vi "InitializeExpDepsFilesWithActualDeps.vi"() -> ()   [LabVIEW 2023, in "Reusables.lvlib"]
uses:
  Reusables/Reusables.lvlib
  <userlib>/_OpenG.lib/file/file.llb/File Exists - Scalar__ogtk.vi
  <userlib>/_OpenG.lib/file/file.llb/openg_file.lvlib
  <vilib>/Utility/config.llb/NI_LVConfig.lvlib
panel:
  out "error out":errorcluster
  in  "Build Specs Folder Path":path=path "E:/sw-deps-monitor/Source/BuildSpecs"
  in  "error in (no error)":errorcluster
  in  "Source Folder Path":path=path "E:/sw-deps-monitor/Source"
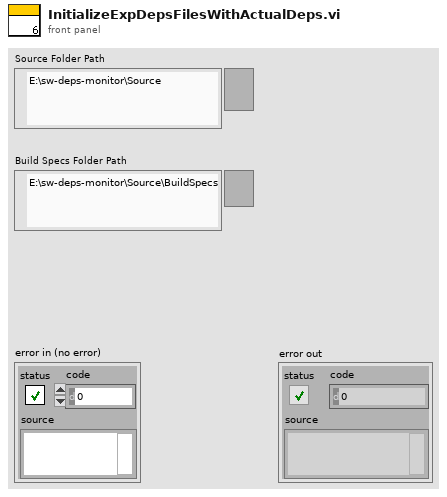
[diagram p1: front panel]
types:
  T1 = typedef "NI_LVConfig.lvlib/Config Data RefNum.ctl" = refnum<k1>
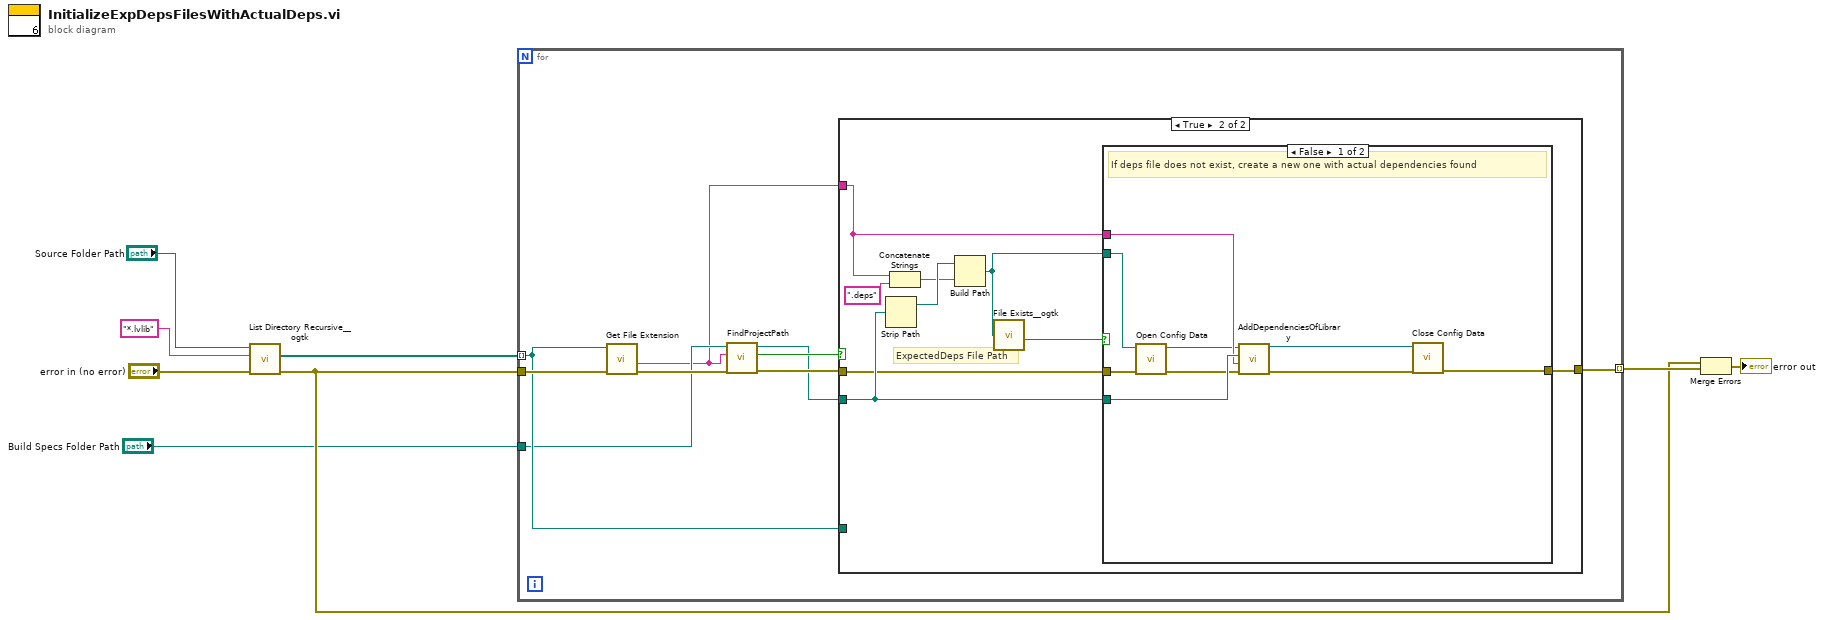
[diagram p0: block diagram]
diagram:
  n1 = call <userlib>:"List Directory Recursive__ogtk.vi"("error in (no error)"="error in (no error)", "pattern"="*.lvlib", "Path"="Source Folder Path") -> ("error out"=w3:errorcluster, "file paths"=w5:path[])  [unwired: 5 in, 2 out]
  n2 = for {
    tunnel: w3 -> [w17]
    tunnel: w5 -> [w15] mode=indexing
    tunnel: "Build Specs Folder Path" -> [w13]
    tunnel: [w16] -> w4 mode=indexing
    n3 = call <vilib>:"Get File Extension.vi"("error in (no error)"=w17, "file"=w15) -> ("error out"=w14:errorcluster, "filename without extension"=w9:string)  [unwired: 5 in, 3 out]
    n4 = call "FindProjectPath.vi"("error in (no error)"=w14, "Library Name"=w9, "Build Specs Folder Path"=w13) -> ("error out"=w11:errorcluster, "Found?"=w12:bool, "Project Path"=w10:path)  [unwired: 6 in]
    n5 = case shown="True" w12 {
      tunnel: w11 -> [w18 w24]
      tunnel: w15 -> [_ _]
      tunnel: [w18 w19] -> w16
      tunnel: w10 -> [_ w27]
      tunnel: w9 -> [_ w20]
      frame False {
      }
      frame True {
        # "ExpectedDeps File Path"
        n6 = Strip Path(path=w27) -> (stripped path=w26:path)  [unwired: 1 out]
        n7 = Concatenate Strings(w20, ".deps" ("string")) -> (w25:string)
        n8 = Build Path(base path=w26, name or relative path=w25) -> (appended path=w22:path)
        n9 = call-poly <userlib>:"File Exists__ogtk.vi"("file path"=w22) -> ("exists"=w21:bool)  [unwired: 6 in, 1 out]
        n10 = case shown="False" w21 {
          tunnel: w27 -> [w36 _]
          tunnel: w24 -> [w35 w37]
          tunnel: w22 -> [w34 _]
          tunnel: w20 -> [w32 _]
          tunnel: [w28 w37] -> w19
          frame False {
            # "If deps file does not exist, create a new one with actual dependencies found"
            n11 = call <vilib>:"Open Config Data.vi"("error in (no error)"=w35, "configuration file path"=w34) -> ("error out"=w33:errorcluster, "refnum"=w31:T1)  [unwired: 7 in, 1 out]
            n12 = call "AddDependenciesOfLibrary.vi"("error in (no error)"=w33, "LibraryName"=w32, "Project Path"=w36, "Config Refnum in"=w31) -> ("error out"=w30:errorcluster, "Config Refnum out"=w29:T1)  [unwired: 6 in]
            n13 = call <vilib>:"Close Config Data.vi"("error in (no error)"=w30, "refnum"=w29) -> ("error out"=w28:errorcluster)  [unwired: 8 in, 1 out]
          }
          frame True {
          }
        }
      }
    }
  }
  n14 = Merge Errors(w3, w4) -> (→"error out":errorcluster)
